vi "Write Scannable.vi"(8 "error in (no error)":errorcluster, 10 "Scannable.lvclass":refnum<class "Scannable.lvclass">, 11 "Scanner.lvclass in":refnum<class "Scanner.lvclass">) -> (0 "error out":errorcluster, 3 "Scanner.lvclass out":refnum<class "Scanner.lvclass">)   [LabVIEW 2012, in "Scanner.lvclass"]
doc: "(Protected) Update the Scannable inside this Scanner instance, after it has been accessed with \"Read Scannable.vi\"."
uses:
  Scanner.lvclass
  Instruments/Utility Classes/Scannable/Scannable.lvclass
  Scanner.lvclass/Scanner.ctl
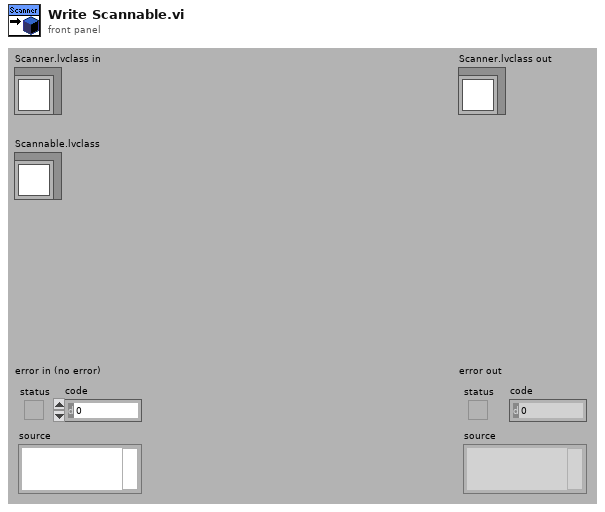
[diagram p1: front panel]
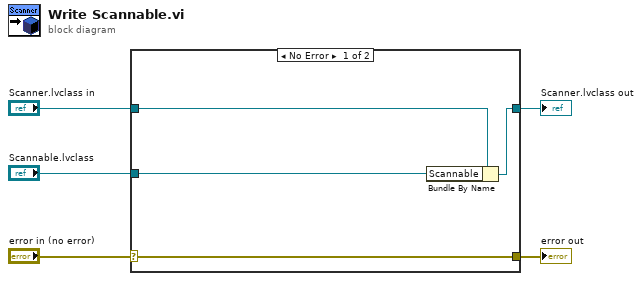
[diagram p0: block diagram]
diagram:
  n1 = case shown="No Error" "error in (no error)" {
    selector: "error in (no error)" -> [w9 w10]
    tunnel: [w9 w10] -> w4
    tunnel: [w7 w11] -> w2
    tunnel: "Scanner.lvclass in" -> [w8 w11]
    tunnel: "Scannable.lvclass" -> [w6 _]
    frame No Error {
      n2 = Bundle By Name(cluster=w8, "Scannable"=w6) -> (w7:refnum<class "Scanner.lvclass">)
    }
    frame Error {
    }
  }
  "error out" <- w4
  "Scanner.lvclass out" <- w2
